vi "Launcher.vi"() -> ()   [LabVIEW 2020]
uses:
  Customer A/Customer A/Customer A.lvclass
  E:/Program Files (x86)/National Instruments/LabVIEW 2020/vi.lib/ActorFramework/Actor/Actor.lvclass
  ShopAssistant/ShopAssistant/ShopAssistant.lvclass
  Customer A/Customer A/Customer A.lvclass/Customer A.ctl
  <vilib>/ActorFramework/Message Enqueuer/Message Enqueuer.lvclass/Message Enqueuer.ctl
  <vilib>/ActorFramework/Message Enqueuer/Enqueue.vi
  Customer A/Customer A Messages/Ask Price Msg/Ask Price Msg.lvclass
  E:/Program Files (x86)/National Instruments/LabVIEW 2020/vi.lib/ActorFramework/Message/Message.lvclass
  Customer A/Customer A Messages/Customer FB Msg/Customer FB Msg.lvclass
  <vilib>/ActorFramework/Stop Msg/Stop Msg.lvclass
  <vilib>/ActorFramework/Message Priority Queue/Priority Enqueue.vi
  <vilib>/ActorFramework/Actor/Actor.lvclass
panel:
  in  "Stop":bool
  in  "Bear Price?":bool
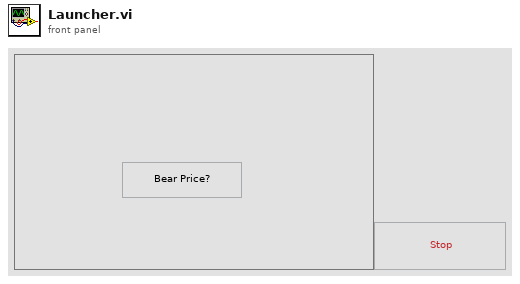
[diagram p1: front panel]
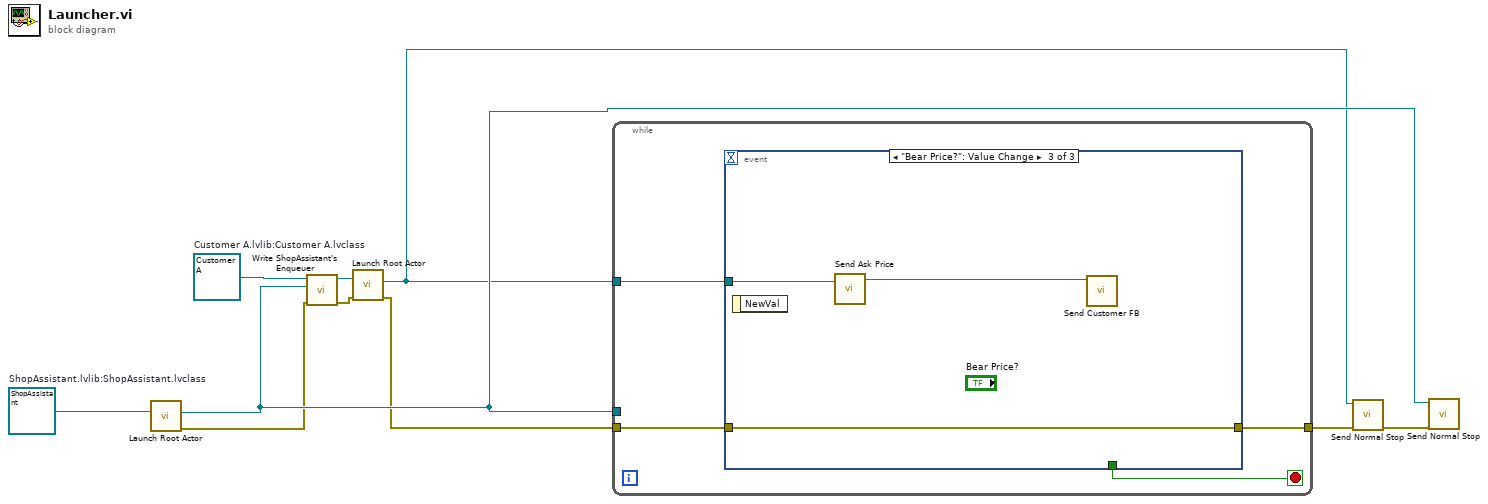
[diagram p0: block diagram]
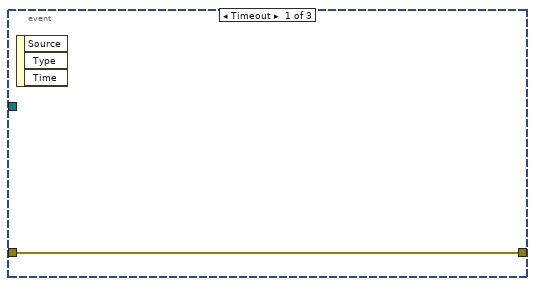
[diagram p2: hidden frame]
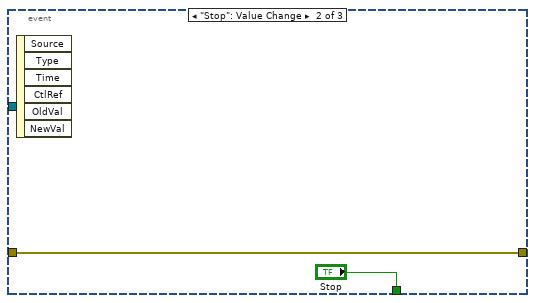
[diagram p3: hidden frame]
diagram:
  w2 = refnum<class "ShopAssistant.lvclass"> refnum  # ShopAssistant.lvlib:ShopAssistant.lvclass
  w8 = refnum<class "Customer A.lvclass"> refnum  # Customer A.lvlib:Customer A.lvclass
  n1 = call <vilib>:"Launch Root Actor.vi"("Actor"=w2) -> ("error out"=w5:errorcluster, "Actor's Enqueuer"=w6:refnum<class "Message Enqueuer.lvclass">)  [unwired: 9 in]
  n2 = call "Write ShopAssistant's Enqueuer.vi"("error in (no error)"=w5, "Actor Framework:Message Enqueuer"=w6, "Customer A in"=w8) -> ("error out"=w4:errorcluster, "Customer A out"=w7:refnum<class "Customer A.lvclass">)  [unwired: 7 in]
  n3 = call <vilib>:"Launch Root Actor.vi"("error in (no error)"=w4, "Actor"=w7) -> ("error out"=w3:errorcluster, "Actor's Enqueuer"=w1:refnum<class "Message Enqueuer.lvclass">)  [unwired: 8 in]
  n4 = while {
    tunnel: w1 -> [w11]
    tunnel: w6 -> [_]
    tunnel: w3 -> [w13]
    tunnel: [w12] -> w10
    stop <- w14 stop-if-true
    n5 = event shown="[2] \"Bear Price?\": Value Change" {
      selector: _ -> [_ _ _]
      dyn-events: _ -> [_ _ _]
      timeout: _ -> [_ _ _]
      tunnel: [_ "Stop" _] -> w14
      tunnel: w13 -> [w15 w16 w20]
      tunnel: [w15 w16 w20] -> w12
      tunnel: w11 -> [_ _ w19]
      event Timeout {
        n6 = event-data() -> ()  [unwired: 1 in, 3 out]
      }
      event "Stop": Value Change {
        n7 = event-data() -> ()  [unwired: 1 in, 6 out]
      }
      event "Bear Price?": Value Change {
        n8 = event-data() -> ()  [unwired: 1 in, 1 out]
        n9 = call "Send Ask Price.vi"("Message Enqueuer"=w19) -> ("Message Enqueuer out"=w18:refnum<class "Message Enqueuer.lvclass">)  [unwired: 9 in, 1 out]
        n10 = call "Send Customer FB.vi"("Message Enqueuer"=w18) -> ()  [unwired: 9 in, 2 out]
      }
    }
  }
  n11 = call <vilib>:"Send Normal Stop.vi"("error in (no error)"=w10, "Message Enqueuer"=w1) -> ("error out"=w9:errorcluster)  [unwired: 9 in]
  n12 = call <vilib>:"Send Normal Stop.vi"("error in (no error)"=w9, "Message Enqueuer"=w6) -> ()  [unwired: 9 in, 1 out]
